vi "Tektronix MSO5X Series Acquire Waveform Measurement.vi"() -> ()   [LabVIEW 2018]
doc: "This example illustrates how to configure and read waveform measurement from the immediate measurement or specified displayed measurement using the following steps:\n\n1. Specify a valid VISA session. \n2. Configure measurement in reference level or in absolute level. \n3. Configure the measurement source and the corresponding parameters.\n4. Run the VI."
uses:
  <instrlib>/Tektronix MSO5X Series/Tektronix MSO5X Series.lvlib
panel:
  in  "stop":bool
  in  "Measurement Source2 (CH2)":string="CH2"
  in  "Measurement Source1 (CH1)":string="CH1"
  in  "Maximum Time (10000ms)":u32=10000
  in  "Measurement Function (49: Amplitude)":i32(ring)=49 items=["Period", "Frequency", "Phase", "Unit Interval", "Data Rate", "Rise Time", "Fall Time", "Rising Slew Rate", "Falling Slew Rate", "High Time", "Low Time", "Positive Pulse Width", "Negative Pulse Width", "Burst Width", "Setup Time", "Hold Time", "Skew", "Delay", "N Periods", "Positive Duty Cycle", "Negative Duty Cycle", "SSC Frequency Deviation", "SSC Modulation Rate", "Time Outside Level", "Jitter Summary", "Time Interval Error", "Random Jitter", "Dual-Dirac Random Jitter", "Non-Periodic Jitter", "Total Jitter@BER", "Deterministic Jitter", "Dual-Dirac Deterministic Jitter", "Periodic Jitter", "Data Dependent Jitter", "Duty Cycle Distortion", "Jitter 2", "Jitter 9", "Sub-Rate Jitter", "F/2 Jitter", "F/4 Jitter", "F/8 Jitter", "Phase Noise", "Eye Width", "Eye Width@BER", "Eye Height", "Eye Height@BER", "Eye High", "Eye Low", "Q-Factor", "Amplitude", "Top", "High", "Base", "Low", "DC Common Mode", "AC Common Mode", "RMS", "AC RMS", "Positive Overshoot", "Negative Overshoot", "Mean", "Area", "Minimum", "Maximum", "V-Diff-Xovr", "Pk-Pk", "T/nT Ratio", "Bit High", "Bit Low", "Bit Amplitude"]
  in  "Measurement Number (1)":i32=1
  out "Measurement Value":dbl
  in  "VISA resource name":refnum<visa-resource-name>
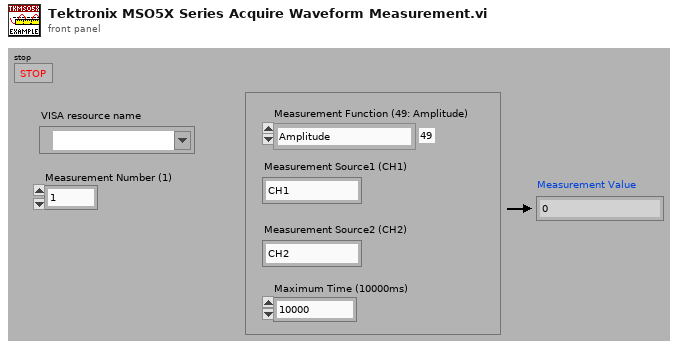
[diagram p1: front panel]
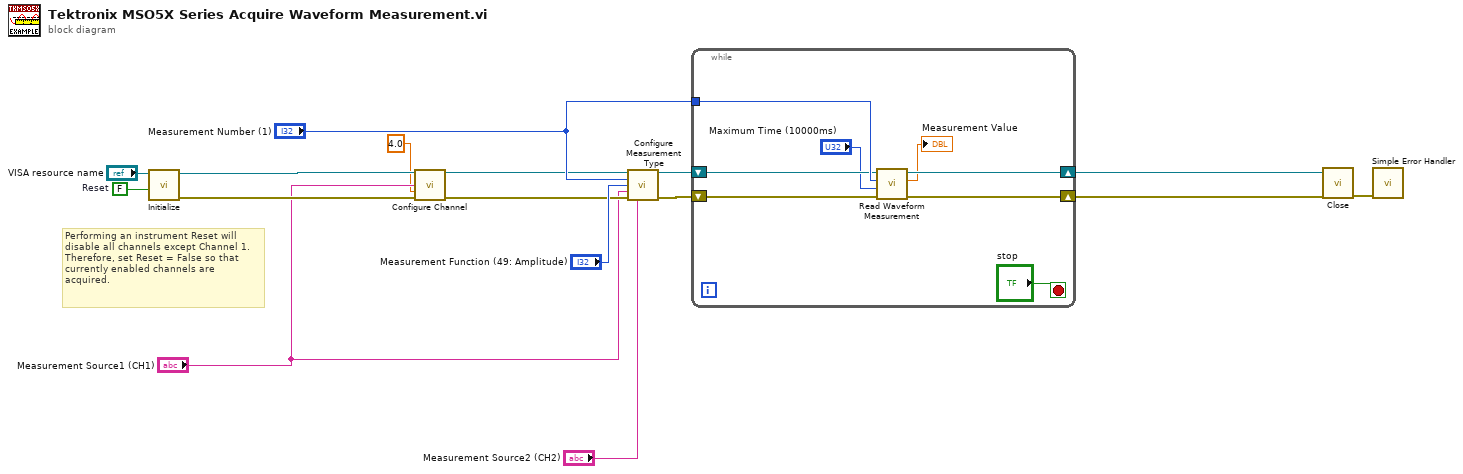
[diagram p0: block diagram]
diagram:
  w14 = FALSE  # Reset
  # "Performing an instrument Reset will disable all channels except Channel 1. Therefore, set Reset = False so that currently enabled channels are acquired."
  n1 = call <instrlib>:"Initialize.vi"("Reset (True)"=w14, "VISA resource name"="VISA resource name") -> ("error out"=w6:errorcluster, "VISA resource name out"=w5:refnum<visa-resource-name>)  [unwired: 8 in]
  n2 = call <instrlib>:"Configure Channel.vi"("VISA resource name"=w5, "Channel (CH1)"="Measurement Source1 (CH1)", "Vertical Range (10.0 V)"=4.0 ("Vertical Offset (0.0 V)"), "error in (no error)"=w6) -> ("VISA resource name out"=w2:refnum<visa-resource-name>, "error out"=w4:errorcluster)  [unwired: 10 in]
  n3 = call <instrlib>:"Configure Measurement Type.vi"("VISA resource name"=w2, "Measurement Number (1)"="Measurement Number (1)", "Measurement Function (0: Period)"="Measurement Function (49: Amplitude)", "Measurement Source1 (CH1)"="Measurement Source1 (CH1)", "error in (no error)"=w4, "Measurement Source2 (CH2)"="Measurement Source2 (CH2)") -> ("VISA resource name out"=w8:refnum<visa-resource-name>, "error out"=w7:errorcluster)  [unwired: 8 in]
  n4 = while {
    tunnel: "Measurement Number (1)" -> [w24]
    shift-right: [w23] -> w12
    shift-left: w8 -> [w21]
    shift-right: [w22] -> w11
    shift-left: w7 -> [w20]
    stop <- "stop" stop-if-true
    n5 = call <instrlib>:"Read Waveform Measurement.vi"("error in (no error)"=w20, "Maximum Time (10000ms)"="Maximum Time (10000ms)", "Measurement Number (1)"=w24, "VISA resource name"=w21) -> ("error out"=w22:errorcluster, "Measurement Value"=→"Measurement Value":dbl, "VISA resource name out"=w23:refnum<visa-resource-name>)  [unwired: 5 in]
  }
  n6 = call <instrlib>:"Close.vi"("error in (no error)"=w11, "VISA resource name"=w12) -> ("error out"=w15:errorcluster)  [unwired: 9 in]
  n7 = call <vilib>:"Simple Error Handler.vi"("error in (no error)"=w15) -> ()  [unwired: 4 in, 5 out]
